vi "Precision Control.vi"(10 "Precision":u8, 11 "Input Value":dbl) -> (2 "Output Value string":string, 3 "Output Value":dbl)   [LabVIEW 2017]
panel:
  # "SUBROUTINE"
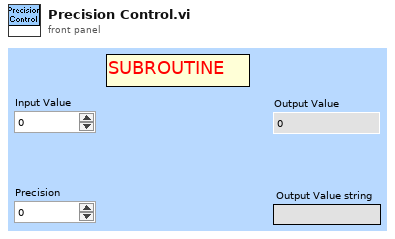
[diagram p1: front panel]
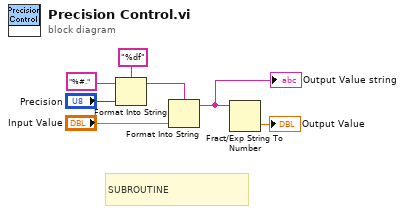
[diagram p0: block diagram]
diagram:
  # "SUBROUTINE"
  n1 = Format Into String(format string="%df", initial string="%#." ("format string"), "Precision") -> (resulting string=w2:string)  [unwired: 1 in, 1 out]
  n2 = Format Into String(format string=w2, "Input Value") -> (resulting string=w3:string)  [unwired: 2 in, 1 out]
  "Output Value string" <- w3
  n3 = Fract/Exp String To Number(string=w3) -> (number=→"Output Value":dbl)  [unwired: 3 in, 1 out]
